vi "CHD_DRIVE_DASH_WRITE.vi"   [LabVIEW 2019]
uses:
  CHD_DRIVE_GLOBALS.vi
  <vilib>/Rock Robotics/Network Tables/NT Write Numeric Array.vi
  <vilib>/Rock Robotics/Network Tables/NT Write Number.vi
  <vilib>/Rock Robotics/WPI/ThirdParty/JAS_Junk/TrajLib/Trajectory_Library.lvlib
types:
  T1 = typedef "Trajectory_Library.lvlib/CHASSIS_SPEEDS.ctl" = cluster{"vX":dbl, "vY":dbl, "vOmega":dbl}
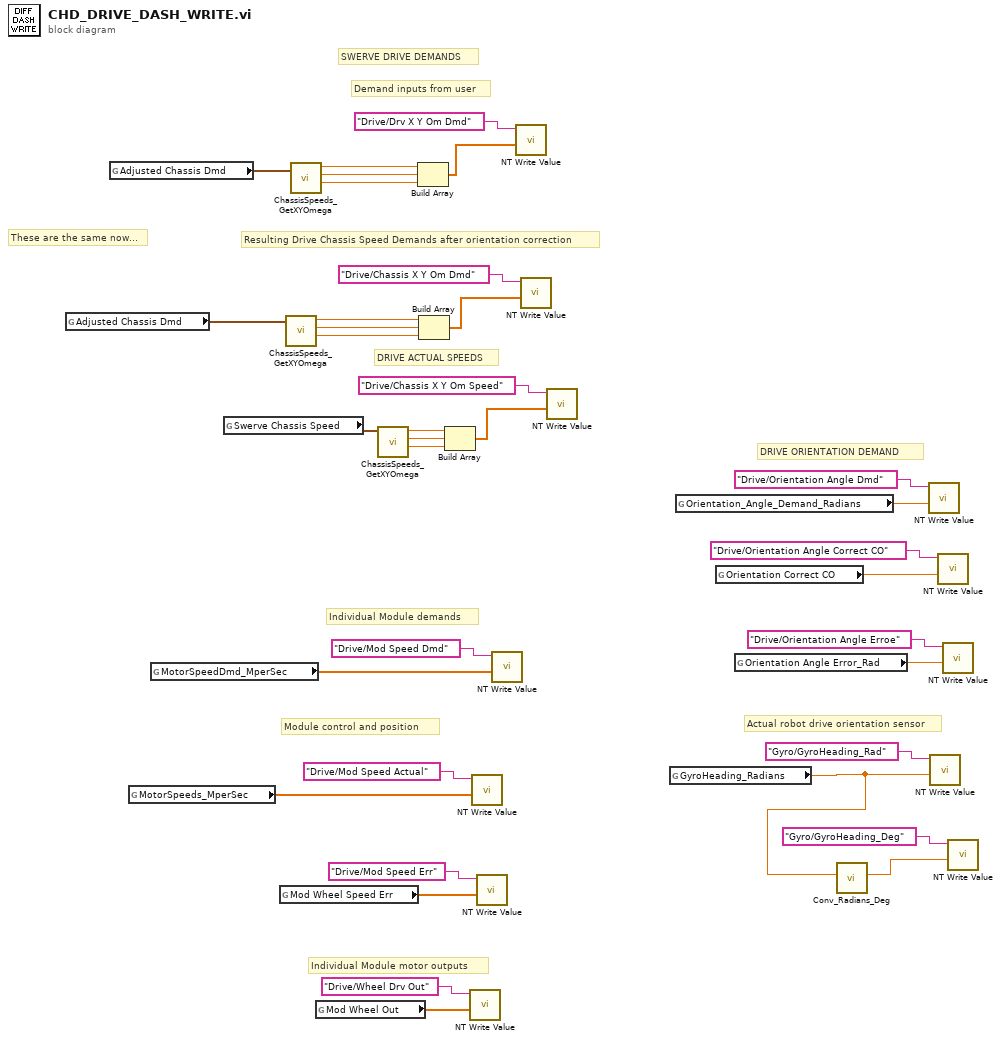
[diagram p0: block diagram]
diagram:
  # "These are the same now..."
  # "Module control and position"
  # "Actual robot drive orientation sensor"
  # "DRIVE ACTUAL SPEEDS"
  # "DRIVE ORIENTATION DEMAND"
  # "Individual Module motor outputs"
  # "Individual Module demands"
  # "Resulting Drive Chassis Speed Demands after orientation correction"
  # "Demand inputs from user"
  # "SWERVE DRIVE DEMANDS"
  n1 = global read "CHD_DRIVE_GLOBALS.vi" "Adjusted Chassis Dmd"() -> (w10:T1)
  n2 = global read "CHD_DRIVE_GLOBALS.vi" "Adjusted Chassis Dmd"() -> (w14:T1)
  n3 = global read "CHD_DRIVE_GLOBALS.vi" "MotorSpeeds_MperSec"() -> (w2:dbl[])
  n4 = global read "CHD_DRIVE_GLOBALS.vi" "MotorSpeedDmd_MperSec"() -> (w1:dbl[])
  n5 = global read "CHD_DRIVE_GLOBALS.vi" "Swerve Chassis Speed"() -> (w6:T1)
  n6 = global read "CHD_DRIVE_GLOBALS.vi" "Mod Wheel Speed Err"() -> (w22:dbl[])
  n7 = call <vilib>:"ChassisSpeeds_GetXYOmega.vi"("CHASSIS"=w10) -> ("vAngular"=w7:dbl, "vY"=w8:dbl, "vX"=w9:dbl)  [unwired: 8 in]
  n8 = call <vilib>:"ChassisSpeeds_GetXYOmega.vi"("CHASSIS"=w14) -> ("vAngular"=w11:dbl, "vY"=w12:dbl, "vX"=w13:dbl)  [unwired: 8 in]
  n9 = global read "CHD_DRIVE_GLOBALS.vi" "Mod Wheel Out"() -> (w21:dbl[])
  n10 = call <vilib>:"ChassisSpeeds_GetXYOmega.vi"("CHASSIS"=w6) -> ("vAngular"=w3:dbl, "vY"=w4:dbl, "vX"=w5:dbl)  [unwired: 8 in]
  n11 = Build Array(w13, w12, w11) -> (w26:dbl[])
  n12 = Build Array(w9, w8, w7) -> (w28:dbl[])
  n13 = Build Array(w5, w4, w3) -> (w33:dbl[])
  n14 = call-poly <vilib>:"NT Write Value.vi"("Numeric Array"=w21, "Name"="Drive/Wheel Drv Out") -> ()  [unwired: 9 in, 1 out]
  n15 = call-poly <vilib>:"NT Write Value.vi"("Numeric Array"=w2, "Name"="Drive/Mod Speed Actual") -> ()  [unwired: 9 in, 1 out]
  n16 = call-poly <vilib>:"NT Write Value.vi"("Numeric Array"=w22, "Name"="Drive/Mod Speed Err") -> ()  [unwired: 9 in, 1 out]
  n17 = call-poly <vilib>:"NT Write Value.vi"("Numeric Array"=w1, "Name"="Drive/Mod Speed Dmd") -> ()  [unwired: 9 in, 1 out]
  n18 = call-poly <vilib>:"NT Write Value.vi"("Numeric Array"=w26, "Name"="Drive/Drv X Y Om Dmd") -> ()  [unwired: 9 in, 1 out]
  n19 = call-poly <vilib>:"NT Write Value.vi"("Numeric Array"=w28, "Name"="Drive/Chassis X Y Om Dmd") -> ()  [unwired: 9 in, 1 out]
  n20 = call-poly <vilib>:"NT Write Value.vi"("Numeric Array"=w33, "Name"="Drive/Chassis X Y Om Speed") -> ()  [unwired: 9 in, 1 out]
  n21 = global read "CHD_DRIVE_GLOBALS.vi" "GyroHeading_Radians"() -> (w15:dbl)
  n22 = global read "CHD_DRIVE_GLOBALS.vi" "Orientation_Angle_Demand_Radians"() -> (w20:dbl)
  n23 = global read "CHD_DRIVE_GLOBALS.vi" "Orientation Correct CO"() -> (w19:dbl)
  n24 = global read "CHD_DRIVE_GLOBALS.vi" "Orientation Angle Error_Rad"() -> (w18:dbl)
  n25 = call <vilib>:"Conv_Radians_Deg.vi"("Radians"=w15) -> ("Degrees"=w16:dbl)  [unwired: 10 in]
  n26 = call-poly <vilib>:"NT Write Value.vi"("Numeric"=w20, "Name"="Drive/Orientation Angle Dmd") -> ()  [unwired: 9 in, 1 out]
  n27 = call-poly <vilib>:"NT Write Value.vi"("Numeric"=w15, "Name"="Gyro/GyroHeading_Rad") -> ()  [unwired: 9 in, 1 out]
  n28 = call-poly <vilib>:"NT Write Value.vi"("Numeric"=w19, "Name"="Drive/Orientation Angle Correct CO") -> ()  [unwired: 9 in, 1 out]
  n29 = call-poly <vilib>:"NT Write Value.vi"("Numeric"=w18, "Name"="Drive/Orientation Angle Erroe") -> ()  [unwired: 9 in, 1 out]
  n30 = call-poly <vilib>:"NT Write Value.vi"("Numeric"=w16, "Name"="Gyro/GyroHeading_Deg") -> ()  [unwired: 9 in, 1 out]
